vi "RFmx Config - PAE.vi"(8 "error in":errorcluster, 10 "RFmx Settings":T1 {"Attenuation"."s2p File"."RFmx S-Parameters Orientation" items=["Port1 Towards DUT"=24000, "Port2 Towards DUT"=24001]; "Attenuation"."Constant Attenuation"."RFmx External Attenuation (dB)" format="%.2f"}, 11 "PAE Reference in":T2) -> (0 "error out":errorcluster, 3 "PAE Reference out":T2)   [LabVIEW 2023]
uses:
  <vilib>/niPAEML/Typedefs/Session Handle.ctl
  <vilib>/niPAEML/PAE Reference.lvclass
  Controls/RFmx Config - Compression.ctl
  FPT Shared VIs/De-embedding/RFmx Config.ctl
  <vilib>/niPAEML/PAE Measurement.lvlib
  <resource>/objmgr/RFmxSpecAn.rc
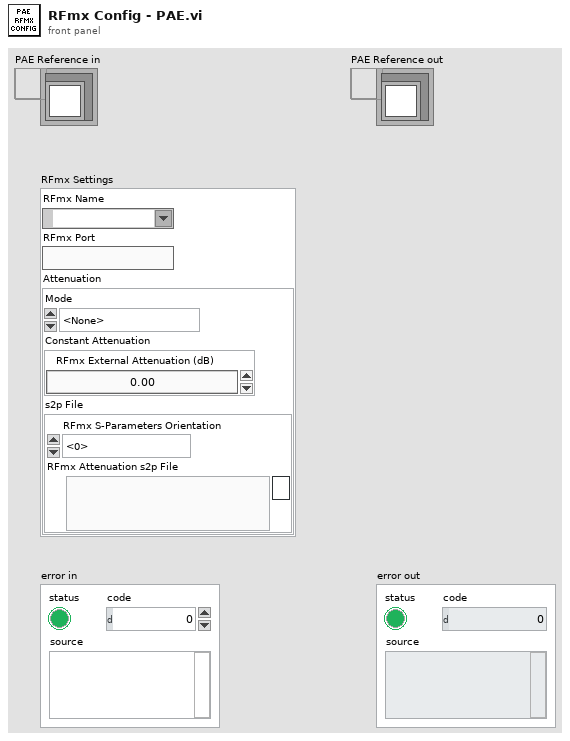
[diagram p1: front panel]
types:
  T1 = typedef "RFmx Config - Compression.ctl" = cluster{"RFmx Name":refnum<k15>, "RFmx Port":string, "Attenuation":cluster{"Mode":enum32{"<None>", "Constant Attenuation", "s2p File"}, "Constant Attenuation":cluster{"RFmx External Attenuation (dB)":dbl}, "s2p File":cluster{"RFmx S-Parameters Orientation":i32, "RFmx Attenuation s2p File":path}}}
  T2 = typedef "PAE Measurement.lvlib/PAE Reference.lvclass/Session Handle.ctl" = refnum<data-value>
  T3 = typedef "RFmx Config.ctl" = cluster{"RFmx Name":refnum<k15>, "RFmx Port":string, "Attenuation":cluster{"Mode":enum32{"<None>", "Constant Attenuation", "s2p File"}, "Constant Attenuation":cluster{"RFmx External Attenuation (dB)":dbl}, "s2p File":cluster{"RFmx S-Parameters Orientation":i32, "RFmx Attenuation s2p Path Name":string, "RFmx Attenuation s2p File":path}}}
  T4 = enum32{"<None>", "Constant Attenuation", "s2p File"}
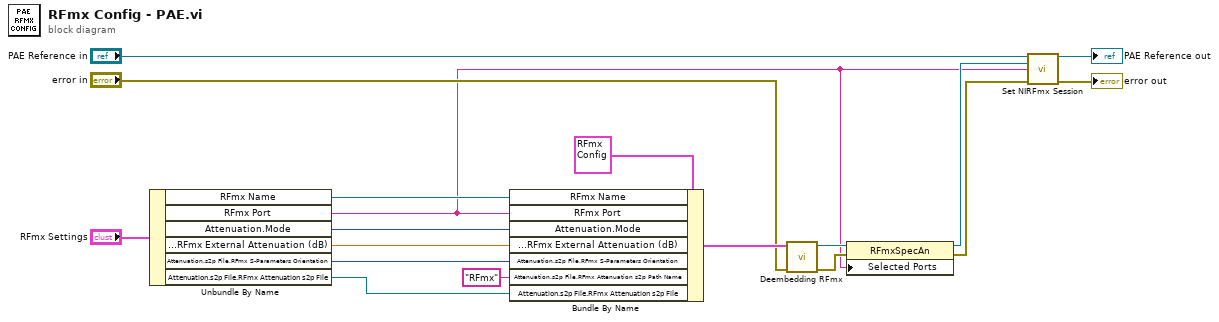
[diagram p0: block diagram]
diagram:
  n1 = Unbundle By Name("RFmx Settings") -> ("RFmx Name"=w11:refnum<k15>, "RFmx Port"=w1:string, "Attenuation.Mode"=w17:T4, "Attenuation.Constant Attenuation.RFmx External Attenuation (dB)"=w14:dbl, "Attenuation.s2p File.RFmx S-Parameters Orientation"=w16:i32, "Attenuation.s2p File.RFmx Attenuation s2p File"=w15:path)
  n2 = Bundle By Name(cluster=T3 {"RFmx Name"="5842_0", "RFmx Port"="", "Attenuation"={"Mode"=enum."Constant Attenuation", "Constant Attenuation"={"RFmx External Attenuation (dB)"=1.2}, "s2p File"={"RFmx S-Parameters Orientation"=24000, "RFmx Attenuation s2p Path Name"="", "RFmx Attenuation s2p File"=path ""}}} ("RFmx Settings"), "RFmx Name"=w11, "RFmx Port"=w1, "Attenuation.Mode"=w17, "Attenuation.Constant Attenuation.RFmx External Attenuation (dB)"=w14, "Attenuation.s2p File.RFmx S-Parameters Orientation"=w16, "Attenuation.s2p File.RFmx Attenuation s2p Path Name"="RFmx", "Attenuation.s2p File.RFmx Attenuation s2p File"=w15) -> (w10:T3)
  n3 = call "Deembedding RFmx.vi"("error in"="error in", "RFmx Settings"=w10) -> ("error out"=w4:errorcluster, "Refnum out"=w5:refnum<k21>)  [unwired: 8 in]
  n4 = property class="RFmxSpecAn"(reference=w5, error in=w4, "Selected Ports"=w1) -> (reference out=w3:refnum<k21>, error out=w2:errorcluster)
  n5 = call <vilib>:"Set NIRFmx Session.vi"("PAE Reference In"="PAE Reference in", "NI RFmx Instrument Handle"=w3, "NI RFmx Port"=w1, "error in"=w2) -> ("PAE Reference Out"=→"PAE Reference out":T2, "error out"=→"error out":errorcluster)  [unwired: 10 in]
